vi "RFID_TAGS_Sort.vi"(11 "TagData in":cluster{"TagCode":string, "FirstSeemUs":u64}[](array[cluster])) -> (2 "TagString":string, 3 "TagArray":string[](array[string]))   [LabVIEW 2015]
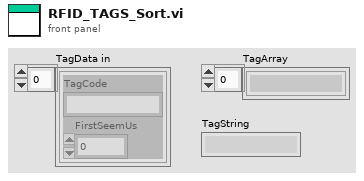
[diagram p1: front panel]
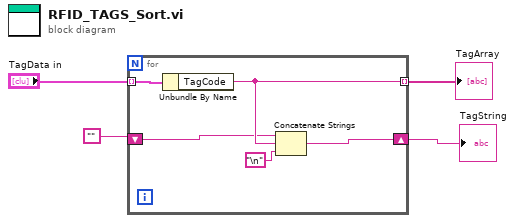
[diagram p0: block diagram]
diagram:
  n1 = for {
    tunnel: "TagData in" -> [w9] mode=indexing
    tunnel: [w7] -> w3 mode=indexing
    shift-right: [w8] -> w4
    shift-left: "" -> [w5]
    n2 = Unbundle By Name(w9) -> ("TagCode"=w7:string)
    n3 = Concatenate Strings(w5, w7, "\n") -> (w8:string)
  }
  "TagArray" <- w3
  "TagString" <- w4
